vi "RefreshTimerPeroid.vi"(8 "error in (no error)":errorcluster, 11 "UserEventTimer in":refnum<class "TimerEngine.lvclass">) -> (0 "error out":errorcluster, 1 "Proper TimePeroid(ms)":i64, 3 "UserEventTimer out":refnum<class "TimerEngine.lvclass">)   [LabVIEW 2017, in "TimerEngine.lvlib" / "TimerEngine.lvclass"]
uses:
  TimerEngine.lvclass
  TimerEngine.lvclass/TimerEngine.ctl
  _TimerClass/Timer.lvclass/Timer.ctl
  _TimerClass/Timer.lvclass
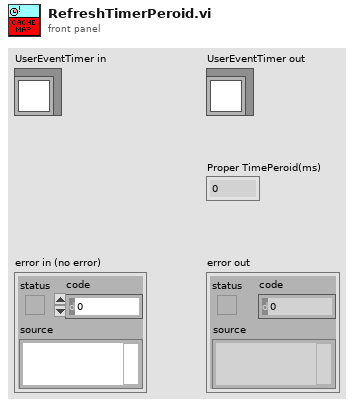
[diagram p1: front panel]
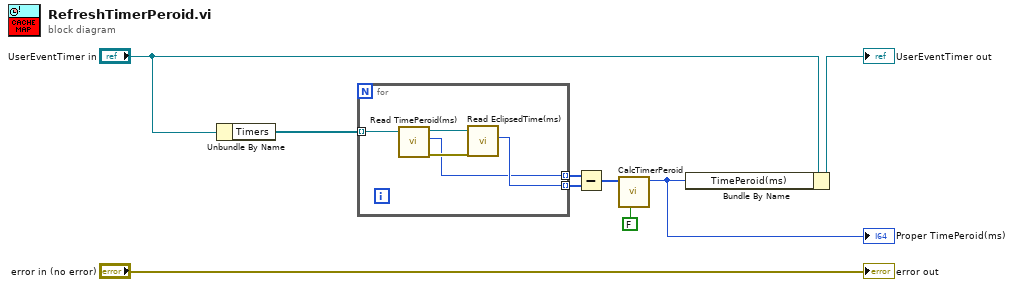
[diagram p0: block diagram]
diagram:
  n1 = Unbundle By Name("UserEventTimer in") -> ("Timers"=w4:refnum<class "Timer.lvclass">[])
  n2 = for {
    tunnel: w4 -> [w14] mode=indexing
    tunnel: [w11] -> w3 mode=indexing
    tunnel: [w10] -> w2 mode=indexing
    n3 = call "Read TimePeroid(ms).vi"("Timer in"=w14) -> ("error out"=w13:errorcluster, "TimePeroid(ms)"=w10:i64, "Timer out"=w12:refnum<class "Timer.lvclass">)  [unwired: 8 in]
    n4 = call "Read EclipsedTime(ms).vi"("error in (no error)"=w13, "Timer in"=w12) -> ("EclipsedTime(ms)"=w11:i64)  [unwired: 7 in, 2 out]
  }
  n5 = Subtract(x=w2, y=w3) -> (x-y=w1:i64[])
  n6 = call "CalcTimerPeroid.vi"("Exclude Inputs?"=FALSE, "TimePeroid"=w1) -> ("Proper TimePeroid(ms)"=w5:i64)  [unwired: 9 in]
  "Proper TimePeroid(ms)" <- w5
  n7 = Bundle By Name(cluster="UserEventTimer in", "TimePeroid(ms)"=w5) -> (→"UserEventTimer out":refnum<class "TimerEngine.lvclass">)
  "error out" <- "error in (no error)"
